vi "drive_target.vi"() -> ()   [LabVIEW 2015]
uses:
  subvi/controls.llb/command.ctl
  <vilib>/Platform/TimedLoop/XDataNode/timing_clust.ctl
  <vilib>/Platform/TimedLoop/XDataNode/nitl_modes.ctl
  <vilib>/Platform/TimedLoop/XDataNode/wakeup.ctl
  subvi/controls.llb/RTFIFO operate.ctl
  subvi/Enum data queue_Ctrls.ctl
  <vilib>/platform/TimedLoop/XDataNode/XDataNode.xnode
  subvi/event data queues.lvlib
  <vilib>/Platform/TimedLoop/XDataNode/XDNodeRunTimeDep.lvlib
panel:
  out "间隔计数":i32
  out "P_N":bool
  out "pulse":bool=TRUE
  out "pulse NO":i32
  out "data":T1
  out "pat":T2
  out "Sin_MODE_RUN state":string
  out "doing":T3(ring)
  out "Boolean array":bool[](array[boolean])
  out "length 2":i32
  out "length":i32
  out "运行":string
  out "state":T3(ring)
  out "exit":bool=TRUE
  in  "variable":T5 {"command" items=["NO_Action", "start", "pause", "resum", "stop", "config"]}
  in  "error in":errorcluster
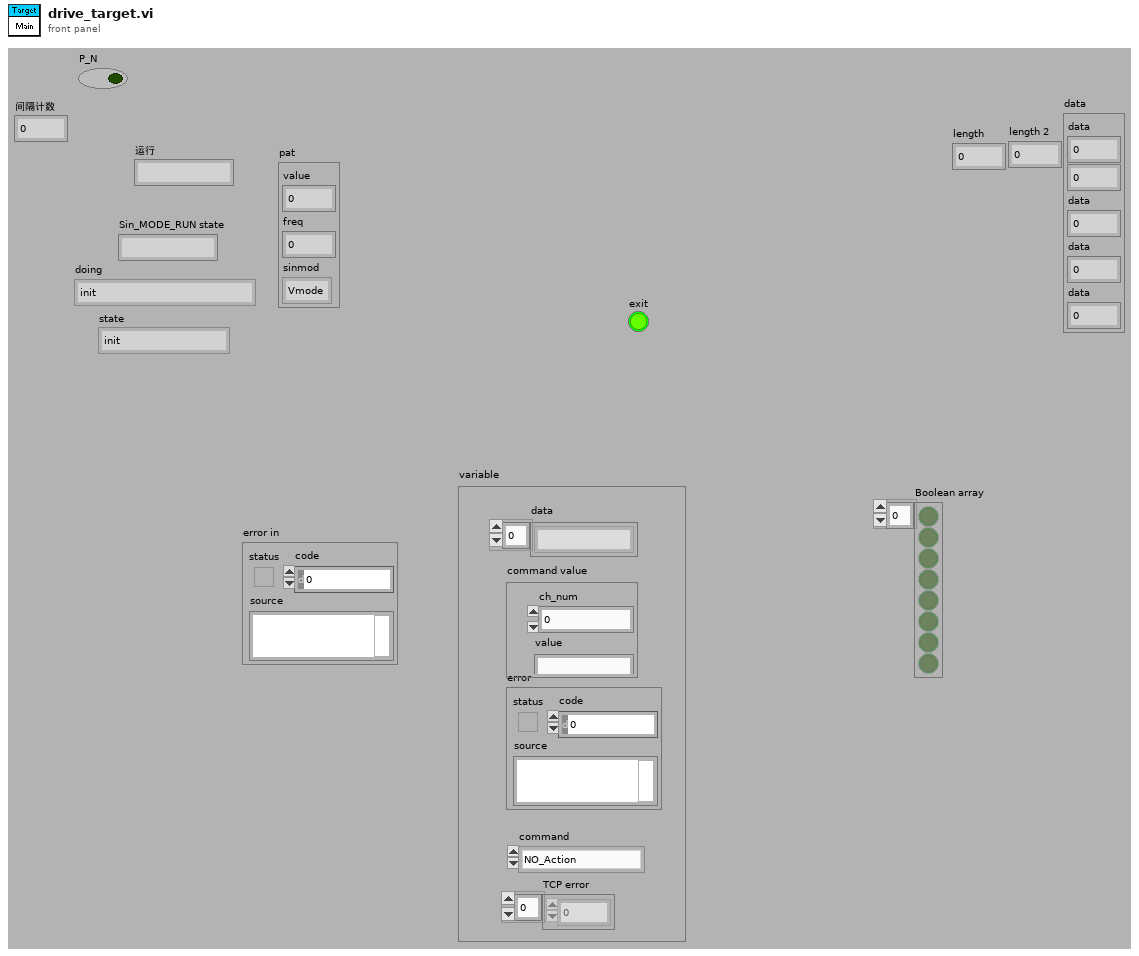
[diagram p1: front panel]
types:
  T1 = cluster{"data":dbl, dbl, "data":u8, "data":dbl, "data":dbl}
  T2 = cluster{"value":dbl, "freq":dbl, "sinmod":enum16{"Vmode", "Tmode", "PConMode", "PNMode"}}
  T3 = enum16{"init", "wait", "start", "do", "stop", "exit"}
  T4 = typedef "command.ctl" = u16
  T5 = cluster{"error":errorcluster, "TCP error":i32[], "command":T4, "command value":cluster{"ch_num":dbl, "value":string}, "data":string[]}
  T6 = typedef "XDNodeRunTimeDep.lvlib/timing_clust.ctl" = cluster{"Expected End [f-1]":u64, "Actual End [f-1]":u64, "Finished Late? [f-1]":bool, "Expected End [i-1]":u64, "Actual End [i-1]":u64, "Finished Late? [i-1]":bool, "Expected Start [i]":u64, "Actual Start [i]":u64, "Expected Start [f]":u64, "Actual Start [f]":u64, "Source Name":string, "Structure Name":string, "Period":i64, "Deadline":i64, "Offset":i64, "Start":i64, "Priority":i32, "Timeout":i32, "Mode":T7, "Wakeup Reason":T8, "Error":errorcluster, "Source Type":string, "Secondary Source Type":string, "Global End Time":u64, "Global Start Time":u64, "Frame Duration":u64, "Iteration Duration":u64, "Assigned CPU":i32, "I/O Scan Engine Mode":u32}
  T7 = typedef "XDNodeRunTimeDep.lvlib/nitl_modes.ctl" = enum32{"No Change", "Process missed periods, maintain original phase", "Discard missed periods, maintain original phase", "Process missed periods, ignore original phase", "Discard missed periods, ignore original phase"}
  T8 = typedef "XDNodeRunTimeDep.lvlib/wakeup.ctl" = enum32{"Normal", "Aborted", "Asynchronous wakeup", "Timing source error", "Timed loop error", "Timeout"}
  T9 = enum16{"init", "config", "start", "write", "stop"}
  T10 = enum16{"init", "config", "start", "read", "stop"}
  T11 = enum16{"connect", "receive data", "send data", "data transfer", "close"}
  T12 = cluster{"data":dbl, "seconds since 1Jan1904":timestamp}
  T13 = enum16{"connect", "receive data", "send data", "data transfer"}
  T14 = typedef "RTFIFO operate.ctl" = enum16{"Creat", "Write", "Read", "Delete"}
  T15 = typedef "event data queues.lvlib/Enum data queue_Ctrls.ctl" = enum16{"Noop", "Send Pro1", "Send data", "Get Pro1", "Get data", "Flush Pro1", "Flush data", "Destroy Pro1", "Destroy data"}
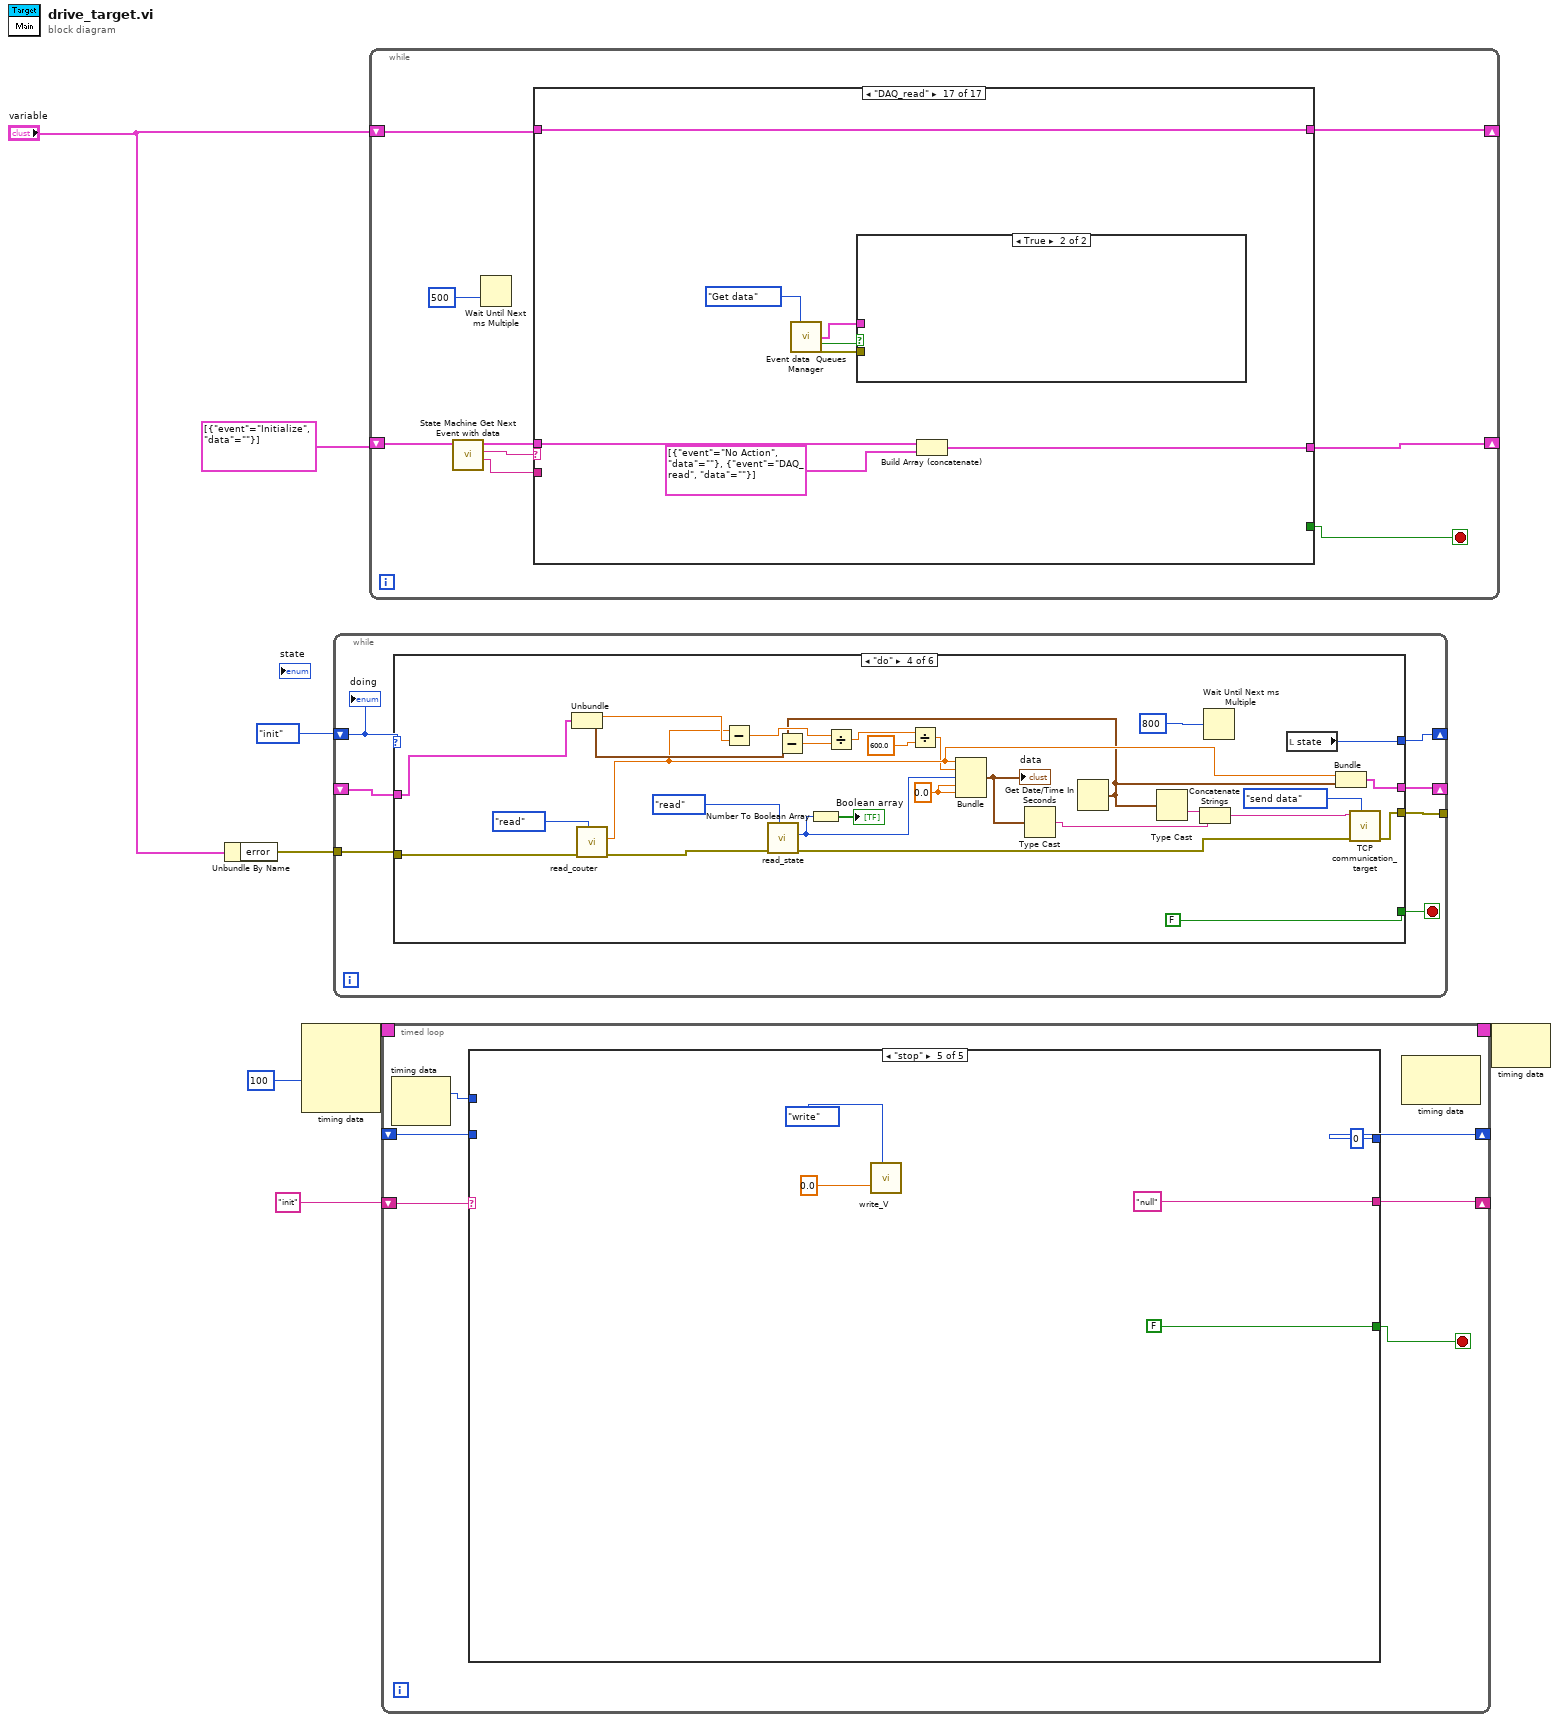
[diagram p0: block diagram]
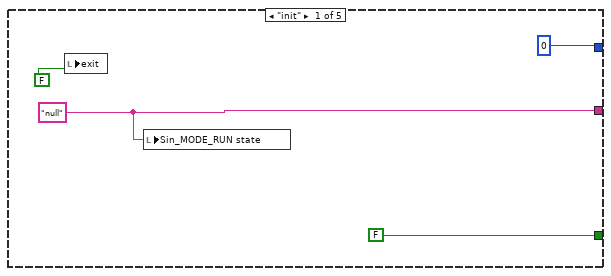
[diagram p2: hidden frame]
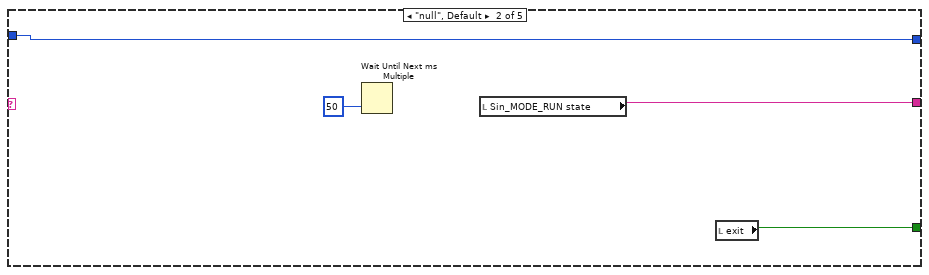
[diagram p3: hidden frame]
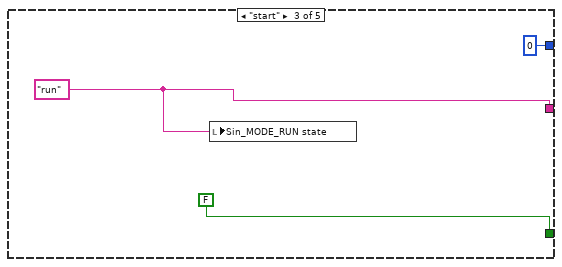
[diagram p4: hidden frame]
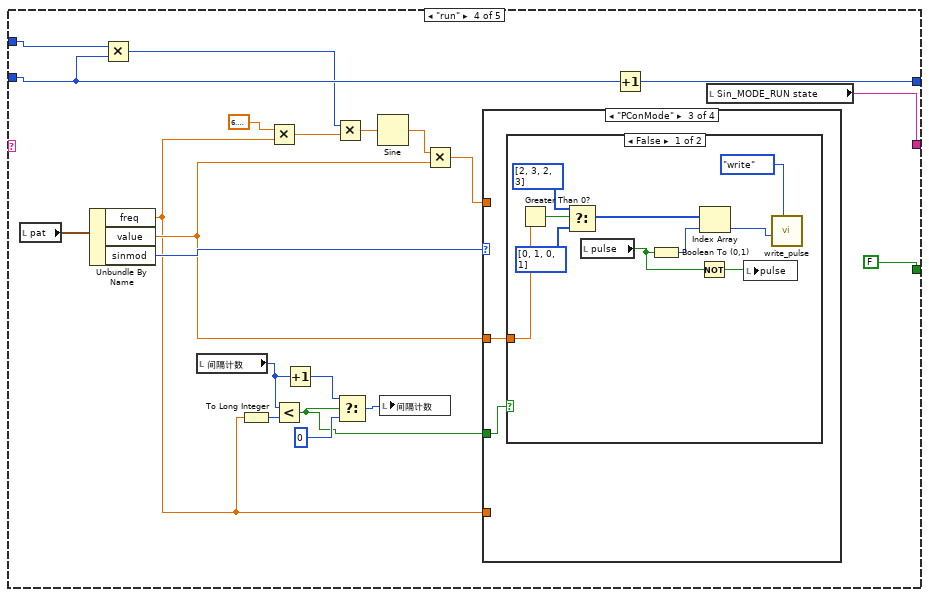
[diagram p5: hidden frame]
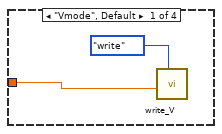
[diagram p6: hidden frame]
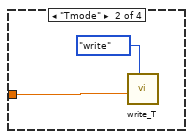
[diagram p7: hidden frame]
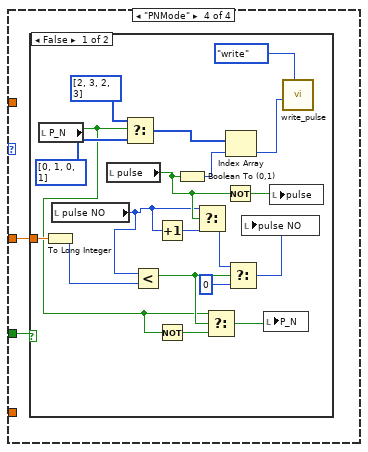
[diagram p9: hidden frame]
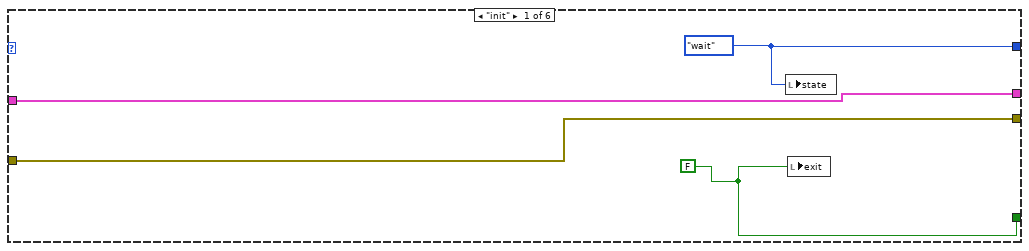
[diagram p11: hidden frame]
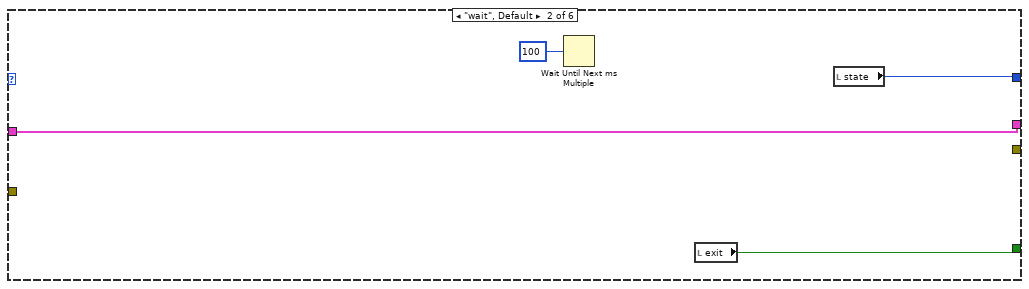
[diagram p12: hidden frame]
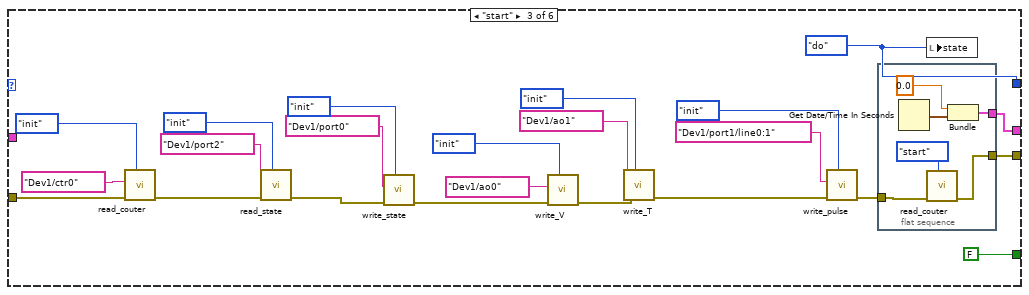
[diagram p13: hidden frame]
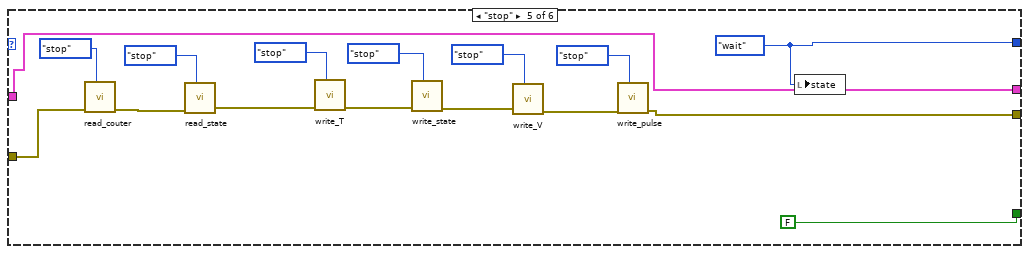
[diagram p14: hidden frame]
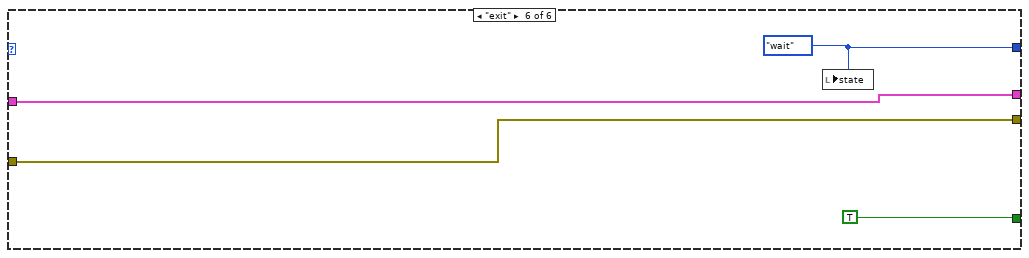
[diagram p15: hidden frame]
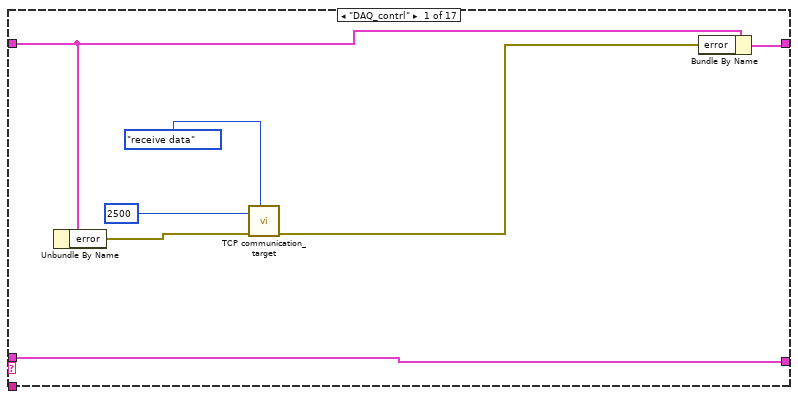
[diagram p16: hidden frame]
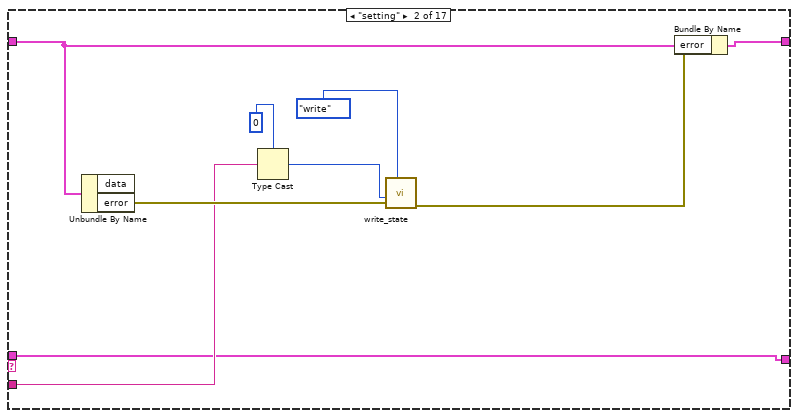
[diagram p17: hidden frame]
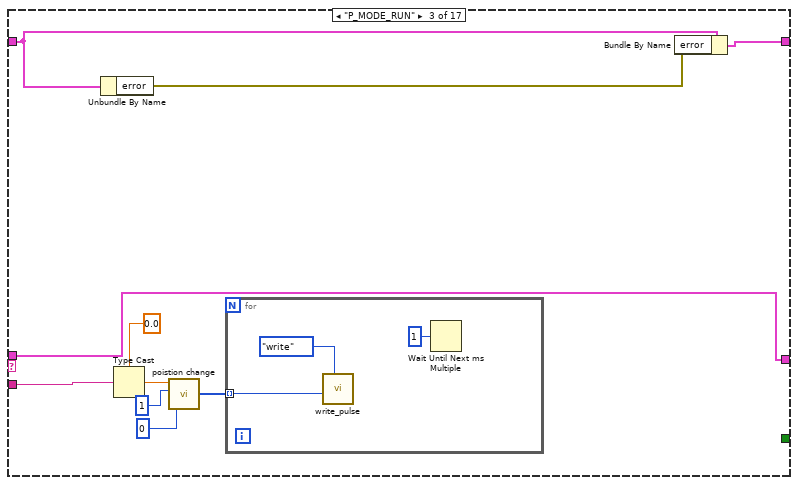
[diagram p18: hidden frame]
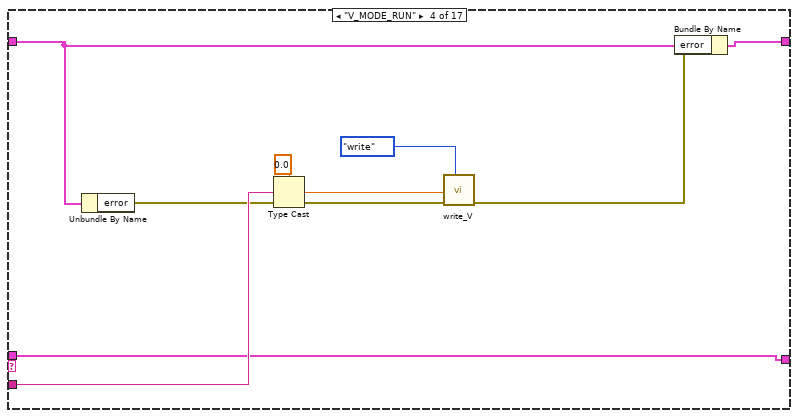
[diagram p19: hidden frame]
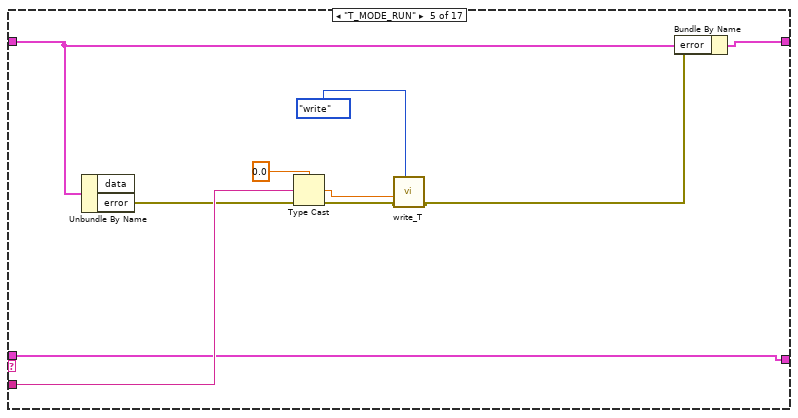
[diagram p20: hidden frame]
diagram:
  n1 = Unbundle By Name("variable") -> ("error"=w7:errorcluster)
  n2 = node-c288(i64 100 ("Period")) -> (w4:T6)  [unwired: 3 in]
  n3 = while {
    shift-right: [w13] -> _
    shift-left: T3."init" ("Enum") -> [w15]
    tunnel: w7 -> [w12]
    tunnel: [w11] -> _
    shift-right: [w10] -> _
    shift-left: _ -> [w9]
    stop <- w14 stop-if-true
    n4 = case shown="\"do\"" w15 {
      tunnel: [w19 w23 FALSE ("exit") FALSE ("exit") FALSE ("exit") TRUE ("exit")] -> w14
      tunnel: [w18 w22 w45 w79 w95 w99] -> w13
      tunnel: w12 -> [w17 _ w41 w78 w94 w98]
      tunnel: [w17 _ w33 w54 w84 w98] -> w11
      tunnel: [w16 w20 w24 w60 w81 w97] -> w10
      tunnel: w9 -> [w16 w20 _ w64 w81 w97]
      frame "init" {
        w18 = T3."wait" ("Enum")
        w19 = FALSE
        n5 = local write "state"(w18) -> ()
        n6 = local write "exit"(w19) -> ()
      }
      frame "wait", Default {
        n7 = Wait Until Next ms Multiple(millisecond multiple=u32 100) -> ()  [unwired: 1 out]
        n8 = local read "exit"() -> (w23:bool)
        n9 = local read "state"() -> (w22:T3)
      }
      frame "start" {
        w45 = T3."do" ("Enum")
        n10 = call "read_couter.vi"("Enum"=T10."init", "error in"=w41, "counter"=tag "Dev1/ctr0") -> ("error out"=w34:errorcluster)  [unwired: 7 in, 1 out]
        n11 = call "read_state.vi"("Enum"=T10."init", "error in"=w34, "lines"=tag "Dev1/port2") -> ("error out"=w40:errorcluster)  [unwired: 7 in, 1 out]
        n12 = call "write_state.vi"("Enum"=T9."init", "error in"=w40, "lines"=tag "Dev1/port0") -> ("error out"=w38:errorcluster)  [unwired: 7 in]
        n13 = call "write_V.vi"("Enum"=T9."init", "error in"=w38, "physical channels"=tag "Dev1/ao0") -> ("error out"=w37:errorcluster)  [unwired: 8 in]
        n14 = call "write_T.vi"("Enum"=T9."init", "error in"=w37, "physical channels"=tag "Dev1/ao1") -> ("error out"=w28:errorcluster)  [unwired: 8 in]
        n15 = call "write_pulse.vi"("Enum"=T9."init", "error in"=w28, "lines"=tag "Dev1/port1/line0:1") -> ("error out"=w27:errorcluster)  [unwired: 7 in]
        n16 = flat-sequence {
          tunnel: [w52] -> w33
          tunnel: w27 -> [w50]
          tunnel: [w49] -> w24
          frame #0 {
            n17 = Get Date/Time In Seconds() -> (seconds since 1Jan1904=w48:timestamp)
            n18 = call "read_couter.vi"("Enum"=T10."start", "error in"=w50) -> ("error out"=w52:errorcluster)  [unwired: 8 in, 1 out]
            n19 = Bundle(0.0, "seconds since 1Jan1904"=w48) -> (w49:cluster{dbl, "seconds since 1Jan1904":timestamp})  [unwired: 1 in]
          }
        }
        n20 = local write "state"(w45) -> ()
      }
      frame "do" {
        w55 = 0.0 ("data")
        n21 = Unbundle(w64) -> ("data"=w62:dbl, "seconds since 1Jan1904"=w63:timestamp)
        n22 = call "read_couter.vi"("Enum"=T10."read", "error in"=w78) -> ("error out"=w77:errorcluster, "data"=w59:dbl)  [unwired: 8 in]
        n23 = Subtract(x=w59, y=w62) -> (x-y=w61:dbl)
        n24 = call "read_state.vi"("Enum"=T10."read", "error in"=w77) -> ("error out"=w67:errorcluster, "data"=w74:u8)  [unwired: 8 in]
        n25 = Number To Boolean Array(number=w74) -> (Boolean array=→"Boolean array":bool[])
        n26 = Get Date/Time In Seconds() -> (seconds since 1Jan1904=w58:timestamp)
        n27 = Subtract(x=w58, y=w63) -> (x-y=w65:dbl)
        n28 = Divide(x=w61, y=w65) -> (x/y=w53:dbl)
        n29 = Divide(x=w53, y=600.0) -> (x/y=w57:dbl)
        n30 = Bundle("data"=w59, w57, "data"=w74, "data"=w55, "data"=w55) -> (w72:T1)  [unwired: 1 in]
        "data" <- w72
        n31 = Type Cast(x=w72) -> (*(type *) &x=w68:string)  [unwired: 1 in]
        n32 = Type Cast(x=w58) -> (*(type *) &x=w66:string)  [unwired: 1 in]
        n33 = Concatenate Strings(w66, w68) -> (w69:string)
        n34 = Wait Until Next ms Multiple(millisecond multiple=u32 800) -> ()  [unwired: 1 out]
        n35 = local read "state"() -> (w79:T3)
        n36 = Bundle("data"=w59, "seconds since 1Jan1904"=w58) -> (w60:T12)  [unwired: 1 in]
        n37 = call "TCP communication_target.vi"("TCP command"=T11."send data", "error in"=w67, "data in"=w69) -> ("error out"=w54:errorcluster)  [unwired: 7 in, 1 out]
      }
      frame "stop" {
        w95 = T3."wait" ("Enum")
        n38 = call "read_couter.vi"("Enum"=T10."stop", "error in"=w94) -> ("error out"=w93:errorcluster)  [unwired: 8 in, 1 out]
        n39 = call "read_state.vi"("Enum"=T10."stop", "error in"=w93) -> ("error out"=w92:errorcluster)  [unwired: 8 in, 1 out]
        n40 = call "write_T.vi"("Enum"=T9."stop", "error in"=w92) -> ("error out"=w91:errorcluster)  [unwired: 9 in]
        n41 = call "write_state.vi"("Enum"=T9."stop", "error in"=w91) -> ("error out"=w86:errorcluster)  [unwired: 8 in]
        n42 = call "write_V.vi"("Enum"=T9."stop", "error in"=w86) -> ("error out"=w85:errorcluster)  [unwired: 9 in]
        n43 = call "write_pulse.vi"("Enum"=T9."stop", "error in"=w85) -> ("error out"=w84:errorcluster)  [unwired: 8 in]
        n44 = local write "state"(w95) -> ()
      }
      frame "exit" {
        w99 = T3."wait" ("Enum")
        n45 = local write "state"(w99) -> ()
      }
    }
    "doing" <- w15
  }
  n46 = while {
    shift-right: [w106] -> _
    shift-left: cluster{"event":string, "data":string}[] [{"event"="Initialize", "data"=""}] ("enent data queue in") -> [w102]
    shift-right: [w104] -> _
    shift-left: "variable" -> [w105]
    stop <- w108 stop-if-true
    n47 = call "State Machine Get Next Event with data.vi"("enent data queue in"=w102) -> ("data"=w101:string, "next event"=w109:string, "event queue out"=w107:cluster{"event":string, "data":string}[])  [unwired: 4 in]
    n48 = Wait Until Next ms Multiple(millisecond multiple=u32 500) -> ()  [unwired: 1 out]
    n49 = case shown="\"DAQ_read\"" w109 {
      selector: w109 -> [_ _ _ _ _ _ _ _ _ _ w207 _ _ _ _ _ _]
      tunnel: [_ _ _ _ _ _ _ _ w194 _ _ _ _ _ _ _ _] -> w108
      tunnel: w107 -> [w114 w117 w126 w139 w148 w162 w172 w180 w193 w206 w209 w262 w270 w272 w277 _ w289]
      tunnel: [w114 w117 w126 w139 w148 w162 w172 w179 w193 w205 w208 w261 w269 w272 w276 w278 w288] -> w106
      tunnel: w105 -> [w112 w123 w135 w147 w156 w161 w173 w182 w192 w202 w212 w266 w268 w271 w274 w281 w287]
      tunnel: [w111 w122 w134 w146 w155 w161 w173 w181 w192 w201 w210 w266 w268 w271 w274 w281 w287] -> w104
      tunnel: w101 -> [_ w118 w132 w144 w153 w164 _ _ _ _ _ _ _ _ _ _ _]
      frame "DAQ_contrl" {
        n50 = Unbundle By Name(w112) -> ("error"=w113:errorcluster)
        n51 = call "TCP communication_target.vi"("TCP command"=T13."receive data", "error in"=w113, "timeout ms"=2500) -> ("error out"=w110:errorcluster)  [unwired: 7 in, 1 out]
        n52 = Bundle By Name(cluster=w112, "error"=w110) -> (w111:T5)
      }
      frame "setting" {
        n53 = Unbundle By Name(w123) -> ("error"=w124:errorcluster)  [unwired: 1 out]
        n54 = Type Cast(type=u8 0, x=w118) -> (*(type *) &x=w119:u8)
        n55 = call "write_state.vi"("Enum"=T9."write", "error in"=w124, "data"=w119) -> ("error out"=w121:errorcluster)  [unwired: 7 in]
        n56 = Bundle By Name(cluster=w123, "error"=w121) -> (w122:T5)
      }
      frame "P_MODE_RUN" {
        n57 = Unbundle By Name(w135) -> ("error"=w131:errorcluster)
        n58 = Type Cast(type=0.0, x=w132) -> (*(type *) &x=w130:dbl)
        n59 = call "poistion change.vi"("Value"=w130, "方向"=u32 1, "位置"=u32 0) -> ("Data"=w127:u8[])  [unwired: 6 in]
        n60 = for {
          tunnel: w127 -> [w137] mode=indexing
          n61 = call "write_pulse.vi"("Enum"=T9."write", "data"=w137) -> ()  [unwired: 8 in, 1 out]
          n62 = Wait Until Next ms Multiple(millisecond multiple=u32 1) -> ()  [unwired: 1 out]
        }
        n63 = Bundle By Name(cluster=w135, "error"=w131) -> (w134:T5)
      }
      frame "V_MODE_RUN" {
        n64 = Unbundle By Name(w147) -> ("error"=w143:errorcluster)
        n65 = Type Cast(type=0.0, x=w144) -> (*(type *) &x=w140:dbl)
        n66 = call "write_V.vi"("Enum"=T9."write", "error in"=w143, "Data"=w140) -> ("error out"=w142:errorcluster)  [unwired: 8 in]
        n67 = Bundle By Name(cluster=w147, "error"=w142) -> (w146:T5)
      }
      frame "T_MODE_RUN" {
        n68 = Unbundle By Name(w156) -> ("error"=w150:errorcluster)  [unwired: 1 out]
        n69 = Type Cast(type=0.0, x=w153) -> (*(type *) &x=w152:dbl)
        n70 = call "write_T.vi"("Enum"=T9."write", "error in"=w150, "Data"=w152) -> ("error out"=w149:errorcluster)  [unwired: 8 in]
        n71 = Bundle By Name(cluster=w156, "error"=w149) -> (w155:T5)
      }
      frame "Sin_MODE_RUN" {
        # "t"
        n72 = Type Cast(type=T2 {"value"=0.0, "freq"=0.0, "sinmod"=enum."Vmode"} ("pat"), x=w164) -> (*(type *) &x=w160:T2)
        "pat" <- w160
        n73 = Unbundle(w160) -> ("value"=w158:dbl, "sinmod"=w159:enum16{"Vmode", "Tmode", "PConMode", "PNMode"})  [unwired: 1 out]
        n74 = case shown="\"PNMode\"" w159 {
          tunnel: w158 -> [_ _ _ _]
          frame "Vmode", Default {
          }
          frame "Tmode" {
          }
          frame "PConMode" {
            n75 = local write "pulse"(FALSE ("pulse")) -> ()
            "间隔计数" <- 0
          }
          frame "PNMode" {
            n76 = local write "间隔计数"(0 ("间隔计数")) -> ()
            "pulse NO" <- 0
            "pulse" <- FALSE
            "P_N" <- TRUE ("P_N")
          }
        }
        "Sin_MODE_RUN state" <- "start"
      }
      frame "Sin_MODE_STOP" {
        n77 = local write "Sin_MODE_RUN state"("stop") -> ()
      }
      frame "Error Handle" {
        n78 = Unbundle By Name(w182) -> ("error.code"=w178:i32)
        n79 = In Range and Coerce(upper limit=67, x=w178, lower limit=62) -> (In Range?=w175:bool)  [unwired: 1 out]
        n80 = case shown="True" w175 {
          tunnel: w182 -> [w185 w189]
          tunnel: [w183 w188] -> w181
          tunnel: [_ cluster{"event":string, "data":string}[] [{"event"="Wait For Connection", "data"=""}] ("array")] -> w174
          frame False {
            n81 = Bundle By Name(cluster=w185, "error"=errorcluster {"status"=FALSE, "code"=0, "source"=""}) -> (w183:T5)
          }
          frame True {
            (unwired) "Wait For Connection"
            # "TCP错误"
            n82 = call "TCP communication_target.vi"("TCP command"=T11."close") -> ()  [unwired: 9 in, 2 out]
            n83 = Bundle By Name(cluster=w189, "error"=errorcluster {"status"=FALSE, "code"=0, "source"=""}) -> (w188:T5)
          }
        }
        n84 = Build Array (concatenate)(w180, w174) -> (w179:cluster{"event":string, "data":string}[])
      }
      frame "Exit" {
        w194 = TRUE
        n85 = local write "state"(T3."exit" ("Enum")) -> ()
        "exit" <- w194
      }
      frame "Initialize" {
        w199 = 66 items=["No Error", "Argument Error", "Memory Full", "Out of Zone", "End of File", "File Already Open", "Generic File IO Error", "File Not Found", "File Permission Error", "Disk Full", "Duplicate Path", "Too Many Files Open", "Not Enabled", "Resource File Not Found", "Cannot Add Resource", "Resource Not Found", "Image Not Found", "Image Memory Error", "Pen Does Not Exist", "Config Bad Type", "Config Token Not Found", "Config Parse Error", "Config Memory Error", "Bad External Code Format", "Bad External Code Offset", "External Code Not Present", "Null Window", "Destroy Window Mixup", "Null Menu", "Print Aborted", "Bad Print Record", "Print Driver Error", "Windows Error During Print", "Memory Error During Print", "Print Dialog Error", "Generic Print Error", "Invalid Device Refnum", "Device Not Found", "Device Parameter Error", "Device Unit Error", "Can't Open Device", "Device Call Aborted", "Generic Error", "Cancelled By User", "Object ID Too Low", "Object ID Too High", "Object Not In Heap", "Unknown Heap", "Bad DefProc ID", "DefProc Not In Table", "Message Out Of Range", "Null Method", "Unknown Message", "Manager Call Not Supported", "Bad address", "Connection In progress", "Connection timed out", "Connection is already in progress", "Network attribute not supported", "Network error", "Address in use", "System out of memory", "Connection aborted", "Connection refused", "Connection is not connected", "Connection is already connected", "Connection closed", "Initialize error (interapplication manager)", "Bad occurrence", "Wait on unbound occurrence handler", "Occurrence queue overflow", "Bad path", "Semaphore not signaled", "Unrecognized type (interapplication manager)"] ("1st Error to Convert")
        w198 = 56 items=["No Error", "Argument Error", "Memory Full", "Out of Zone", "End of File", "File Already Open", "Generic File IO Error", "File Not Found", "File Permission Error", "Disk Full", "Duplicate Path", "Too Many Files Open", "Not Enabled", "Resource File Not Found", "Cannot Add Resource", "Resource Not Found", "Image Not Found", "Image Memory Error", "Pen Does Not Exist", "Config Bad Type", "Config Token Not Found", "Config Parse Error", "Config Memory Error", "Bad External Code Format", "Bad External Code Offset", "External Code Not Present", "Null Window", "Destroy Window Mixup", "Null Menu", "Print Aborted", "Bad Print Record", "Print Driver Error", "Windows Error During Print", "Memory Error During Print", "Print Dialog Error", "Generic Print Error", "Invalid Device Refnum", "Device Not Found", "Device Parameter Error", "Device Unit Error", "Can't Open Device", "Device Call Aborted", "Generic Error", "Cancelled By User", "Object ID Too Low", "Object ID Too High", "Object Not In Heap", "Unknown Heap", "Bad DefProc ID", "DefProc Not In Table", "Message Out Of Range", "Null Method", "Unknown Message", "Manager Call Not Supported", "Bad address", "Connection In progress", "Connection timed out", "Connection is already in progress", "Network attribute not supported", "Network error", "Address in use", "System out of memory", "Connection aborted", "Connection refused", "Connection is not connected", "Connection is already connected", "Connection closed", "Initialize error (interapplication manager)", "Bad occurrence", "Wait on unbound occurrence handler", "Occurrence queue overflow", "Bad path", "Semaphore not signaled", "Unrecognized type (interapplication manager)"] ("1st Error to Convert")
        w200 = 64 items=["No Error", "Argument Error", "Memory Full", "Out of Zone", "End of File", "File Already Open", "Generic File IO Error", "File Not Found", "File Permission Error", "Disk Full", "Duplicate Path", "Too Many Files Open", "Not Enabled", "Resource File Not Found", "Cannot Add Resource", "Resource Not Found", "Image Not Found", "Image Memory Error", "Pen Does Not Exist", "Config Bad Type", "Config Token Not Found", "Config Parse Error", "Config Memory Error", "Bad External Code Format", "Bad External Code Offset", "External Code Not Present", "Null Window", "Destroy Window Mixup", "Null Menu", "Print Aborted", "Bad Print Record", "Print Driver Error", "Windows Error During Print", "Memory Error During Print", "Print Dialog Error", "Generic Print Error", "Invalid Device Refnum", "Device Not Found", "Device Parameter Error", "Device Unit Error", "Can't Open Device", "Device Call Aborted", "Generic Error", "Cancelled By User", "Object ID Too Low", "Object ID Too High", "Object Not In Heap", "Unknown Heap", "Bad DefProc ID", "DefProc Not In Table", "Message Out Of Range", "Null Method", "Unknown Message", "Manager Call Not Supported", "Bad address", "Connection In progress", "Connection timed out", "Connection is already in progress", "Network attribute not supported", "Network error", "Address in use", "System out of memory", "Connection aborted", "Connection refused", "Connection is not connected", "Connection is already connected", "Connection closed", "Initialize error (interapplication manager)", "Bad occurrence", "Wait on unbound occurrence handler", "Occurrence queue overflow", "Bad path", "Semaphore not signaled", "Unrecognized type (interapplication manager)"] ("1st Error to Convert")
        (unwired) "Wait For Connection"
        n86 = Build Array (concatenate)(w206, cluster{"event":string, "data":string} {"event"="Wait For Connection", "data"=""} ("enent data queue in")) -> (w205:cluster{"event":string, "data":string}[])
        n87 = Build Array(w200, w199, w198) -> (w197:i32[])
        n88 = call "RTFIFO Model.vi"("size"=4000, "operate"=RTFIFO_operate."Creat") -> ("error out"=w196:errorcluster)  [unwired: 8 in, 1 out]
        n89 = Bundle By Name(cluster=w202, "TCP error"=w197, "error"=w196) -> (w201:T5)
      }
      frame "Default", Default {
        n90 = Unbundle By Name(w212) -> ("error.status"=w211:bool)
        n91 = case shown="False" w211 {
          tunnel: [w221 w254] -> w210
          tunnel: w212 -> [w220 w254]
          tunnel: w209 -> [w219 w253]
          tunnel: [w218 w252] -> w208
          frame False {
            n92 = call "TCP communication_target.vi"("TCP command"=T13."receive data", "timeout ms"=300) -> ("error out"=w216:errorcluster, "Data out"=w217:string[])  [unwired: 8 in]
            n93 = Unbundle By Name(w216) -> ("code"=w215:i32)
            n94 = Equal?(x=w215, y=56) -> (x = y?=w213:bool)
            n95 = case shown="True" w213 {
              tunnel: [w235 w250] -> w221
              tunnel: w220 -> [w234 w250]
              tunnel: w219 -> [w230 w249]
              tunnel: [w229 w249] -> w218
              tunnel: w217 -> [w226 _]
              tunnel: w216 -> [w227 _]
              frame False {
                n96 = call "convert tcp data (host command).vi"("error in"=w227, "TCP Data"=w226) -> ("error out"=w233:errorcluster, "command"=w228:T4)  [unwired: 8 in]
                n97 = Index Array "Index Array"(array=w226, index=1) -> (element=w224:string)
                n98 = call "case according to command.vi"("error in"=w233, "command"=w228) -> ("error out"=w232:errorcluster, "case"=w231:string)  [unwired: 8 in]
                n99 = case shown="0, Default" w228 {
                  tunnel: w230 -> [w241 w248]
                  tunnel: [w240 w246] -> w229
                  tunnel: w231 -> [w237 w245]
                  tunnel: w224 -> [w236 w242]
                  frame 0, Default {
                    n100 = Bundle By Name(cluster=cluster{"event":string, "data":string} {"event"="", "data"=""} ("new element/subarray"), "event"=w237, "data"=w236) -> (w239:cluster{"event":string, "data":string})
                    n101 = Build Array (concatenate)(w241, w239) -> (w240:cluster{"event":string, "data":string}[])
                  }
                  frame 13 {
                    n102 = Bundle By Name(cluster=cluster{"event":string, "data":string} {"event"="", "data"=""} ("new element/subarray"), "event"=w245, "data"=w242) -> (w243:cluster{"event":string, "data":string})
                    n103 = Insert Into Array "Insert Into Array"(array=w248, index=0, new element=w243) -> (w246:cluster{"event":string, "data":string}[])
                  }
                }
                n104 = Bundle By Name(cluster=w234, "data"=w226, "command"=w228, "error"=w232) -> (w235:T5)
              }
              frame True {
              }
            }
          }
          frame True {
            # "DAQ_read"
            n105 = Build Array (concatenate)(w253, cluster{"event":string, "data":string} {"event"="Error Handle", "data"=""} ("enent data queue in")) -> (w252:cluster{"event":string, "data":string}[])
          }
        }
        "运行" <- w207
      }
      frame "Wait For Connection" {
        n106 = call "TCP communication_target.vi"("TCP command"=T13."connect", "error in"="error in", "remote port"=u16 6342) -> ("error out"=w263:errorcluster)  [unwired: 7 in, 1 out]
        n107 = Select(t="Wait For Connection", s=w263, f="Default") -> (s? t:f=w256:string)
        n108 = Bundle By Name(cluster=cluster{"event":string, "data":string} {"event"="", "data"=""} ("new element/subarray"), "event"=w256) -> (w258:cluster{"event":string, "data":string})
        n109 = Build Array (concatenate)(w262, w258) -> (w261:cluster{"event":string, "data":string}[])
      }
      frame "DAQ_init" {
        n110 = Build Array (concatenate)(w270, cluster{"event":string, "data":string} {"event"="DAQ_config", "data"=""} ("new element/subarray")) -> (w269:cluster{"event":string, "data":string}[])
      }
      frame "DAQ_config" {
      }
      frame "DAQ_start" {
        n111 = local write "state"(T3."start" ("Enum")) -> ()
        n112 = Build Array (concatenate)(w277, cluster{"event":string, "data":string} {"event"="DAQ_read", "data"=""} ("new element/subarray")) -> (w276:cluster{"event":string, "data":string}[])
      }
      frame "DAQ_stop" {
        n113 = local write "state"(T3."stop" ("Enum")) -> ()
        n114 = Build Array(cluster{"event":string, "data":string} {"event"="Default", "data"=""} ("new element/subarray")) -> (w278:cluster{"event":string, "data":string}[])
      }
      frame "DAQ_read" {
        n115 = call "Event data  Queues Manager.vi"("Mode"=Enum_data_queue_Ctrls."Get data") -> ("data"=w283:cluster{"time":timestamp, "data":string}, "timed out?"=w282:bool, "error out"=w284:errorcluster)  [unwired: 11 in, 1 out]
        n116 = case shown="True" w282 {
          tunnel: w284 -> [w297 _]
          tunnel: w283 -> [w296 _]
          frame False {
            n117 = Unbundle By Name(w296) -> ("time"=w295:timestamp, "data"=w290:string)
            n118 = Type Cast(x=w295) -> (*(type *) &x=w291:string)  [unwired: 1 in]
            n119 = String Length(string=w291) -> (length=→"length":i32)
            n120 = String Length(string=w290) -> (length=→"length 2":i32)
            n121 = Concatenate Strings(w291, w290) -> (w294:string)
            n122 = call "TCP communication_target.vi"("TCP command"=T11."send data", "error in"=w297, "data in"=w294) -> ()  [unwired: 7 in, 2 out]
          }
          frame True {
          }
        }
        n123 = Build Array (concatenate)(w289, cluster{"event":string, "data":string}[] [{"event"="No Action", "data"=""}, {"event"="DAQ_read", "data"=""}]) -> (w288:cluster{"event":string, "data":string}[])
      }
    }
  }
  n124 = timed-loop {
    timing: w4 -> [_]
    timing-out: [_] -> w3
    shift-right: [w302] -> _
    shift-left: "init" -> [w304]
    shift-right: [w301] -> _
    shift-left: _ -> [w300]
    stop <- w303 stop-if-true
    n125 = node-c288() -> (w299:i64)  [unwired: 1 in, 1 out]
    n126 = case shown="\"stop\"" w304 {
      tunnel: [FALSE ("exit") w312 FALSE ("exit") FALSE ("exit") FALSE ("exit")] -> w303
      tunnel: [w307 w311 w314 w335 "null" ("Sin_MODE_RUN state")] -> w302
      tunnel: [i64 0 w310 i64 0 w319 i64 0] -> w301
      tunnel: w300 -> [_ w310 _ w317 _]
      tunnel: w299 -> [_ _ _ w318 _]
      frame "init" {
        w307 = "null"
        n127 = local write "exit"(FALSE) -> ()
        n128 = local write "Sin_MODE_RUN state"(w307) -> ()
      }
      frame "null", Default {
        n129 = Wait Until Next ms Multiple(millisecond multiple=u32 50) -> ()  [unwired: 1 out]
        n130 = local read "Sin_MODE_RUN state"() -> (w311:string)
        n131 = local read "exit"() -> (w312:bool)
      }
      frame "start" {
        w314 = "run"
        n132 = local write "Sin_MODE_RUN state"(w314) -> ()
      }
      frame "run" {
        n133 = local read "pat"() -> (w329:T2)
        n134 = Unbundle By Name(w329) -> ("freq"=w326:dbl, "value"=w327:dbl, "sinmod"=w328:enum16{"Vmode", "Tmode", "PConMode", "PNMode"})
        n135 = Multiply(x=w318, y=w317) -> (x*y=w316:i64)
        n136 = local read "间隔计数"() -> (w320:i32)
        n137 = To Long Integer(number=w326) -> (32bit integer=w325:i32)
        n138 = Multiply(x=6.283185307179586, y=w326) -> (x*y=w333:dbl)
        n139 = Less?(x=w320, y=w325) -> (x < y?=w321:bool)
        n140 = Increment(x=w320) -> (x+1=w323:i32)
        n141 = Multiply(x=w316, y=w333) -> (x*y=w332:dbl)
        n142 = Select(t=w323, s=w321, f=0) -> (s? t:f=w322:i32)
        n143 = Sine(x=w332) -> (sin(x)=w331:dbl)
        n144 = local write "间隔计数"(w322) -> ()
        n145 = Multiply(x=w331, y=w327) -> (x*y=w330:dbl)
        n146 = case shown="\"PConMode\"" w328 {
          tunnel: w330 -> [w337 w339 _ _]
          tunnel: w327 -> [_ _ w342 w354]
          tunnel: w326 -> [_ _ _ _]
          tunnel: w321 -> [_ _ w341 w353]
          frame "Vmode", Default {
            n147 = call "write_V.vi"("Enum"=T9."write", "Data"=w337) -> ()  [unwired: 9 in, 1 out]
          }
          frame "Tmode" {
            n148 = call "write_T.vi"("Enum"=T9."write", "Data"=w339) -> ()  [unwired: 9 in, 1 out]
          }
          frame "PConMode" {
            n149 = case shown="False" w341 {
              tunnel: w342 -> [w352 _]
              frame False {
                n150 = Greater Than 0?(x=w352) -> (x > 0?=w351:bool)
                n151 = Select(t=u8[] [2, 3, 2, 3] ("Data"), s=w351, f=u8[] [0, 1, 0, 1] ("Data")) -> (s? t:f=w347:u8[])
                n152 = local read "pulse"() -> (w344:bool)
                n153 = Boolean To (0,1)(Boolean=w344) -> (0, 1=w346:i16)
                n154 = Not(x=w344) -> (.not. x?=w343:bool)
                n155 = Index Array(array=w347, index=w346) -> (element=w345:u8)
                n156 = local write "pulse"(w343) -> ()
                n157 = call "write_pulse.vi"("Enum"=T9."write", "data"=w345) -> ()  [unwired: 8 in, 1 out]
              }
              frame True {
              }
            }
          }
          frame "PNMode" {
            n158 = case shown="False" w353 {
              tunnel: w354 -> [w363 _]
              frame False {
                n159 = local read "P_N"() -> (w356:bool)
                n160 = To Long Integer(number=w363) -> (32bit integer=w362:i32)
                n161 = local read "pulse NO"() -> (w364:i32)
                n162 = local read "pulse"() -> (w366:bool)
                n163 = Select(t=u8[] [2, 3, 2, 3] ("Data"), s=w356, f=u8[] [0, 1, 0, 1] ("Data")) -> (s? t:f=w368:u8[])
                n164 = Less?(x=w364, y=w362) -> (x < y?=w358:bool)
                n165 = Increment(x=w364) -> (x+1=w365:i32)
                n166 = Not(x=w356) -> (.not. x?=w357:bool)
                n167 = Boolean To (0,1)(Boolean=w366) -> (0, 1=w370:i16)
                n168 = Select(t=w364, s=w366, f=w365) -> (s? t:f=w361:i32)
                n169 = Select(t=w356, s=w358, f=w357) -> (s? t:f=w355:bool)
                n170 = Not(x=w366) -> (.not. x?=w369:bool)
                n171 = Index Array(array=w368, index=w370) -> (element=w367:u8)
                n172 = Select(t=w361, s=w358, f=0) -> (s? t:f=w360:i32)
                n173 = local write "pulse NO"(w360) -> ()
                n174 = local write "P_N"(w355) -> ()
                n175 = local write "pulse"(w369) -> ()
                n176 = call "write_pulse.vi"("Enum"=T9."write", "data"=w367) -> ()  [unwired: 8 in, 1 out]
              }
              frame True {
              }
            }
          }
        }
        n177 = Increment(x=w317) -> (x+1=w319:i64)
        n178 = local read "Sin_MODE_RUN state"() -> (w335:string)
      }
      frame "stop" {
        n179 = call "write_V.vi"("Enum"=T9."write", "Data"=0.0) -> ()  [unwired: 9 in, 1 out]
      }
    }
    n180 = node-c288() -> ()  [unwired: 2 in, 1 out]
  }
  n181 = node-c288(w3) -> ()  [unwired: 1 out]
